vi "220613 SD TABLE AVG.vi"(3 "Table of SD to average":dbl[][](array[numeric])) -> (1 "Average SD":dbl[](array[numeric]))   [LabVIEW 2021]
panel:
  out "element 2":i32
  out "element":i32
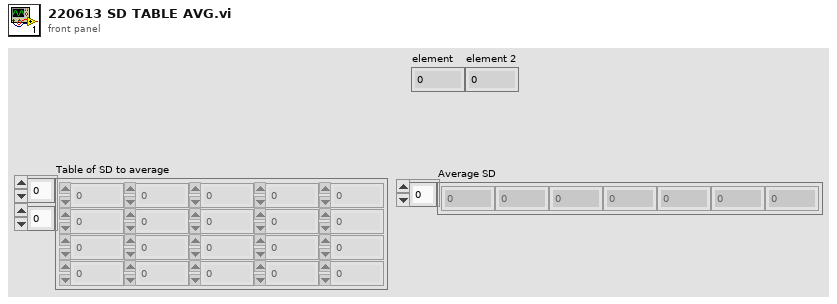
[diagram p1: front panel]
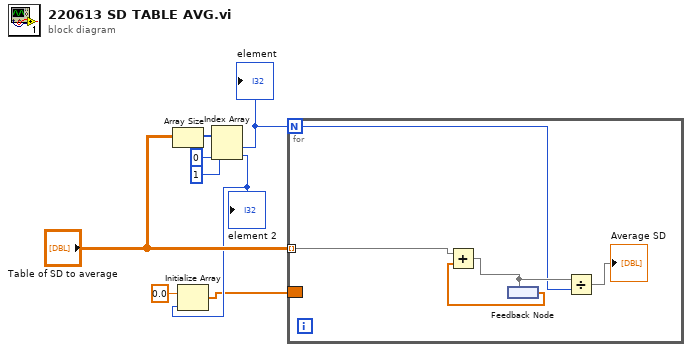
[diagram p0: block diagram]
diagram:
  n1 = Array Size(array="Table of SD to average") -> (size(s)=w7:i32[])
  n2 = Index Array(array=w7, index #1=0 ("index"), index #2=1 ("index")) -> (element #1=w4:i32, element #2=w2:i32)
  "element" <- w4
  "element 2" <- w2
  n3 = Initialize Array(0.0 ("element"), w2) -> (w1:dbl[])
  n4 = for {
    N: w4 -> [w9]
    tunnel: "Table of SD to average" -> [w12] mode=indexing
    border: w1 -> [_]
    n5 = feedback #1() -> (w13:dbl[])
    n6 = Add(x=w12, y=w13) -> (x+y=w11:dbl[])
    n7 = feedback-in #1(w11) -> ()
    n8 = Divide(x=w11, y=w9) -> (x/y=→"Average SD":dbl[])
  }
